vi "Check if Buses Defined.vi"(8 "error in":errorcluster, 11 "Number of Buses":i32) -> (0 "error out":errorcluster)   [LabVIEW 2014, in "SPI Engine Scripting.lvlib"]
doc: "If the number of buses is 0, throw an error because there is nothing to script."
uses:
  SPI Engine Scripting.lvlib
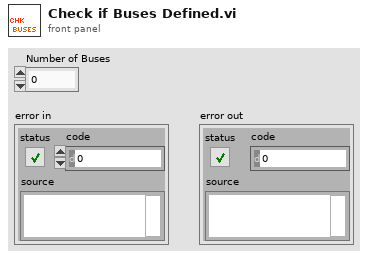
[diagram p1: front panel]
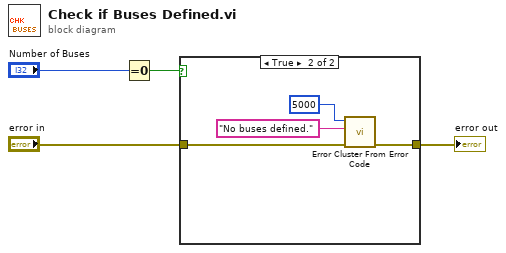
[diagram p0: block diagram]
diagram:
  n1 = Equal To 0?(x="Number of Buses") -> (x = 0?=w1:bool)
  n2 = case shown="True" w1 {
    tunnel: "error in" -> [w5 w9]
    tunnel: [w5 w8] -> w4
    frame False {
    }
    frame True {
      n3 = call <vilib>:"Error Cluster From Error Code.vi"("error in (no error)"=w9, "error message (\"\")"="No buses defined." ("error message (\"\")"), "error code (0)"=5000) -> ("error out"=w8:errorcluster)  [unwired: 6 in]
    }
  }
  "error out" <- w4
